vi "Tell.vi"(10 "Msg":refnum<class "Msg.lvclass">, 11 "Event Transport in":refnum<class "Event Transport.lvclass">) -> (0 "Error out":errorcluster)   [LabVIEW 2025, in "jettl.lvlib" / "Transport.lvlib" / "Event.lvlib" / "Event Transport.lvclass"]
uses:
  Event Transport.lvclass
  Msg/Msg.lvclass
  Event Transport.lvclass/Event Transport.ctl
  <vilib>/event_ctls.llb/usereventprio.ctl
  Teller/Teller.lvclass
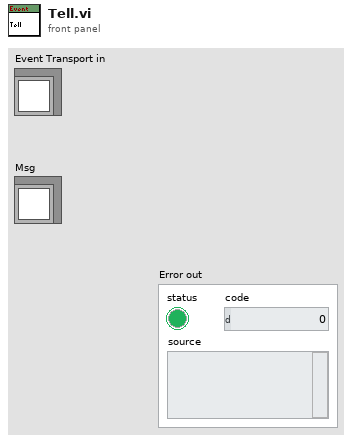
[diagram p1: front panel]
types:
  T1 = typedef "usereventprio.ctl" = enum32{"high priority", "normal priority"}
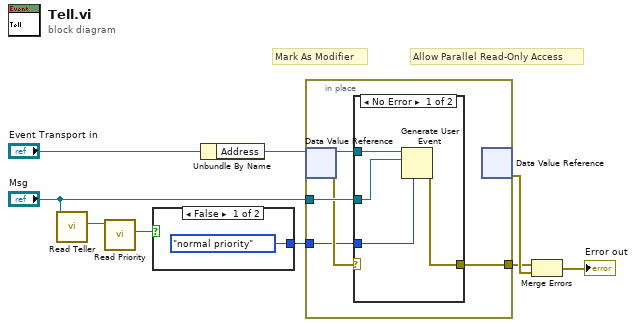
[diagram p0: block diagram]
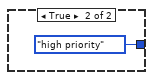
[diagram p3: hidden frame]
diagram:
  # "Allow Parallel Read-Only Access"
  # "Mark As Modifier"
  n1 = call-dynamic "Read Teller.vi"("Msg in"="Msg") -> ("Teller"=w1:refnum<class "Teller.lvclass">)  [unwired: 10 in]
  n2 = call-dynamic "Read Priority.vi"("Teller in"=w1) -> ("Priority"=w3:bool)  [unwired: 10 in]
  n3 = case shown="False" w3 {
    tunnel: [usereventprio."normal priority" ("priority (normal)") usereventprio."high priority" ("priority (normal)")] -> w5
    frame False {
    }
    frame True {
    }
  }
  n4 = Unbundle By Name("Event Transport in") -> ("Address"=w6:refnum<data-value>)
  n5 = in-place {
    in-place-border: [w16] -> w7
    in-place-border: "Msg" -> [w15]
    in-place-border: w5 -> [w12]
    n6 = in-place-dvr #1(w6) -> (w14:refnum<user-event>, w13:errorcluster)
    n7 = case shown="No Error" w13 {
      selector: w13 -> [_ w21]
      tunnel: [w18 w21] -> w16
      tunnel: w15 -> [w19 _]
      tunnel: w14 -> [w20 _]
      tunnel: w12 -> [w17 _]
      frame No Error {
        n8 = Generate User Event(priority (normal)=w17, user event=w20, event data cluster=w19) -> (error out=w18:errorcluster)  [unwired: 1 in, 1 out]
      }
      frame Error {
      }
    }
    n9 = in-place-dvr #1() -> (w8:errorcluster)  [unwired: 1 in, 1 out]
  }
  n10 = Merge Errors(w7, w8) -> (→"Error out":errorcluster)
